vi "Test Decompose and Recompose.vi"() -> ()   [LabVIEW 2026, in "VILab.lvlib"]
uses:
  VILab.lvlib
  CTLs/Resource.ctl
  SubVIs/Decompose VI (Refnum).vi
panel:
  out "Target path out":path
  out "VI Load Result":errorcluster
  out "array of clusters":T2(array[cluster])
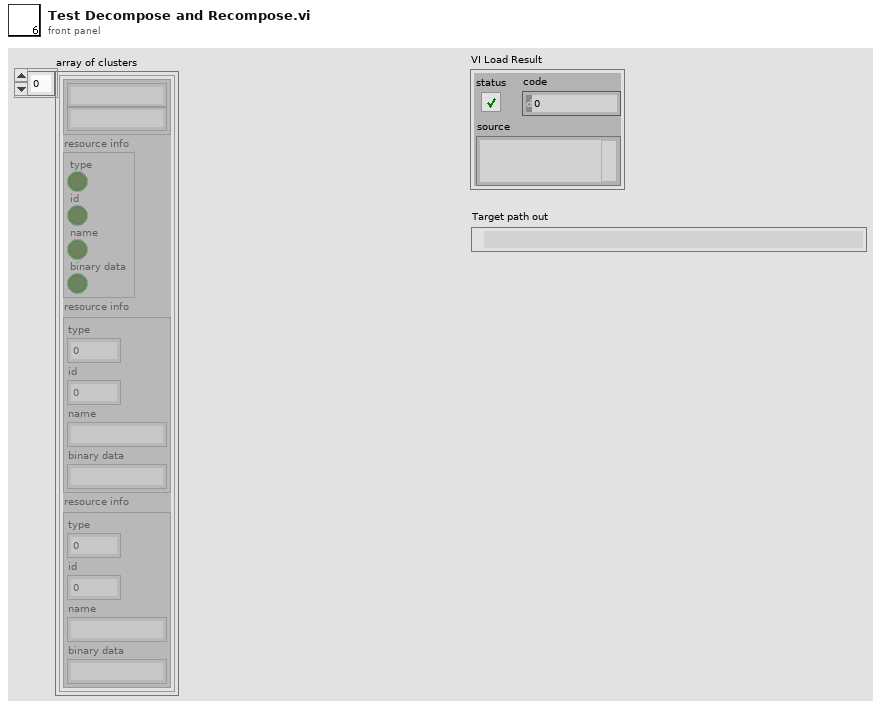
[diagram p1: front panel]
types:
  T1 = typedef "VILab.lvlib/Resource.ctl" = cluster{"type":u32, "id":i32, "name":string, "binary data":string}
  T2 = cluster{cluster{string, string}, "resource info":cluster{"type":bool, "id":bool, "name":bool, "binary data":bool}, "resource info":T1, "resource info":T1}[]
  T3 = cluster{"type":bool, "id":bool, "name":bool, "binary data":bool}[]
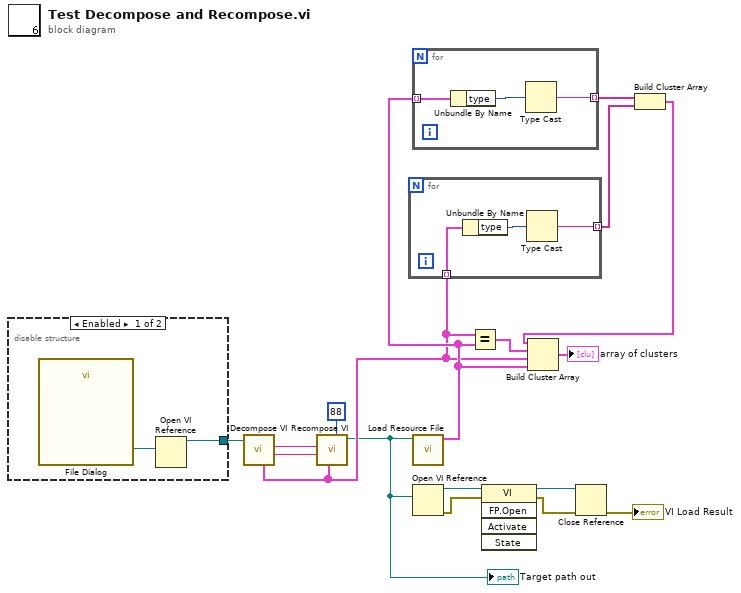
[diagram p0: block diagram]
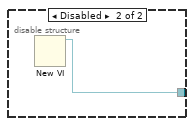
[diagram p2: hidden frame]
diagram:
  n1 = disable-structure shown="Enabled" {
    disable-tunnel: [w18 w20] -> w15
    frame Enabled {
      n2 = call "File Dialog"() -> ("selected path"=w19:path)  [unwired: 12 in, 3 out]
      n3 = Open VI Reference(vi path=w19) -> (vi reference=w18:refnum<vi>)  [unwired: 5 in, 1 out]
    }
    frame Disabled {
      n4 = New VI() -> (3:w20:refnum<vi>)  [unwired: 7 in, 1 out]
    }
  }
  n5 = call-poly "Decompose VI.vi"("VI Ref"=w15) -> ("Block Diagram XML"=w17:string, "Front Panel XML"=w1:string, "Other resources"=w8:T1[])  [unwired: 6 in, 2 out]
  n6 = call "Recompose VI.vi"("FPH_/BDH_ (88=X)"=u8 88, "Other resources (default)"=w8, "Block Diagram XML"=w17, "Front Panel XML"=w1) -> ("Target path out"=w7:path)  [unwired: 5 in, 2 out]
  "Target path out" <- w7
  n7 = for {
    tunnel: w8 -> [w23] mode=indexing
    tunnel: [w21] -> w11 mode=indexing
    n8 = Unbundle By Name(w23) -> ("type"=w22:u32)
    n9 = Type Cast(x=w22) -> (*(type *) &x=w21:string)  [unwired: 1 in]
  }
  n10 = call "Load Resource File.vi"("Resource File"=w7) -> ("Resources"=w13:T1[])  [unwired: 8 in, 2 out]
  n11 = for {
    tunnel: w13 -> [w26] mode=indexing
    tunnel: [w24] -> w12 mode=indexing
    n12 = Unbundle By Name(w26) -> ("type"=w25:u32)
    n13 = Type Cast(x=w25) -> (*(type *) &x=w24:string)  [unwired: 1 in]
  }
  n14 = Open VI Reference(vi path=w7) -> (vi reference=w6:refnum<vi>, error out=w5:errorcluster)  [unwired: 5 in]
  n15 = Equal?(x=w8, y=w13) -> (x = y?=w14:T3)
  n16 = invoke class="VI" method="FP.Open"(reference=w6, error in=w5) -> (reference out=w4:refnum<vi>, error out=w3:errorcluster)  [unwired: 3 in, 3 out]
  n17 = Close Reference(reference=w4, error in (no error)=w3) -> (error out=→"VI Load Result":errorcluster)
  n18 = Build Cluster Array(w12, w11) -> (w10:cluster{string, string}[])
  n19 = Build Cluster Array(w10, w14, w8, w13) -> (→"array of clusters":T2)
